vi "RT Main.vi"() -> ()   [LabVIEW 2015]
uses:
  Controls/RT controls.ctl
panel:
  in  "Under":bool
  in  "Break":bool
  in  "Enum":enum16{"3rd", "2nd", "1st", "N", "R"}(ring)=enum."R"
  in  "Right":bool
  in  "Left":bool
  in  "Headlights":bool
  in  "Gas":bool
  in  "Keyin":bool
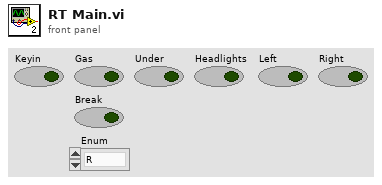
[diagram p1: front panel]
types:
  T1 = typedef "RT controls.ctl" = cluster{"PWM width":dbl, "Headlights":bool, "Red Lights":bool, "Left Turn Lights":bool, "Steer Position":dbl, "Right Turn Lights":bool, "Under Lights":bool}
  T2 = typedef "DIO.lvlib/DIO Reference.ctl" = cluster{"myRIO Reference":T3, "DIO Channels List":T7}
  T3 = typedef "myRIO Generic Hardware Reference.ctl" = cluster{"myRIO Model":T4, "myRIO Hardware Reference":T5}
  T4 = typedef "Hardware Version Enum.ctl" = enum16{"Unknown", "myRIO-1900", "myRIO-1950", "roboRIO"}
  T5 = typedef "myRIO v1.0 Reference.ctl" = cluster{"Generic FPGA Reference":T6, "Allow multiple opens":bool}
  T6 = typedef "Generic FPGA Reference.ctl" = refnum<k20>
  T7 = typedef "DIO Channels List.ctl" = T8[]
  T8 = typedef "DIO Channels Enum.ctl" = enum16{"Not Connected", "C/DIO0", "C/DIO1", "C/DIO2", "C/DIO3", "C/DIO4", "C/DIO5", "C/DIO6", "C/DIO7", "A/DIO0", "A/DIO1", "A/DIO2", "A/DIO3", "A/DIO4", "A/DIO5", "A/DIO6", "A/DIO7", "A/DIO8", "A/DIO9", "A/DIO10", "A/DIO11", "A/DIO12", "A/DIO13", "A/DIO14", "A/DIO15", "B/DIO0", "B/DIO1", "B/DIO2", "B/DIO3", "B/DIO4", "B/DIO5", "B/DIO6", "B/DIO7", "B/DIO8", "B/DIO9", "B/DIO10", "B/DIO11", "B/DIO12", "B/DIO13", "B/DIO14", "B/DIO15", "LED0", "LED1", "LED2", "LED3", "Button0", "DIO/DIO0", "DIO/DIO1", "DIO/DIO2", "DIO/DIO3", "DIO/DIO4", "DIO/DIO5", "DIO/DIO6", "DIO/DIO7", "DIO/DIO8", "DIO/DIO9", "SPI/CS0", "SPI/CS1", "SPI/CS2", "SPI/CS3", "LED RADIO (Green)", "LED RADIO (Red)", "LED COMM (Green)", "LED COMM (Red)", "LED MODE (Green)", "LED MODE (Red)"}
  T9 = typedef "PWM.lvlib/PWM Reference.ctl" = cluster{"myRIO Reference":T3, "PWM Channels Enum":T10, "PWM Configuration":T11}
  T10 = typedef "PWM Channels Enum.ctl" = enum16{"Not Connected", "C/PWM0", "C/PWM1", "A/PWM0", "A/PWM1", "A/PWM2", "B/PWM0", "B/PWM1", "B/PWM2", "PWM/PWM0", "PWM/PWM1", "PWM/PWM2", "PWM/PWM3", "PWM/PWM4", "PWM/PWM5", "PWM/PWM6", "PWM/PWM7", "PWM/PWM8", "PWM/PWM9"}
  T11 = typedef "PWM.lvlib/PWM Configuration.ctl" = cluster{"Frequency":dbl, "Duty Cycle":dbl}
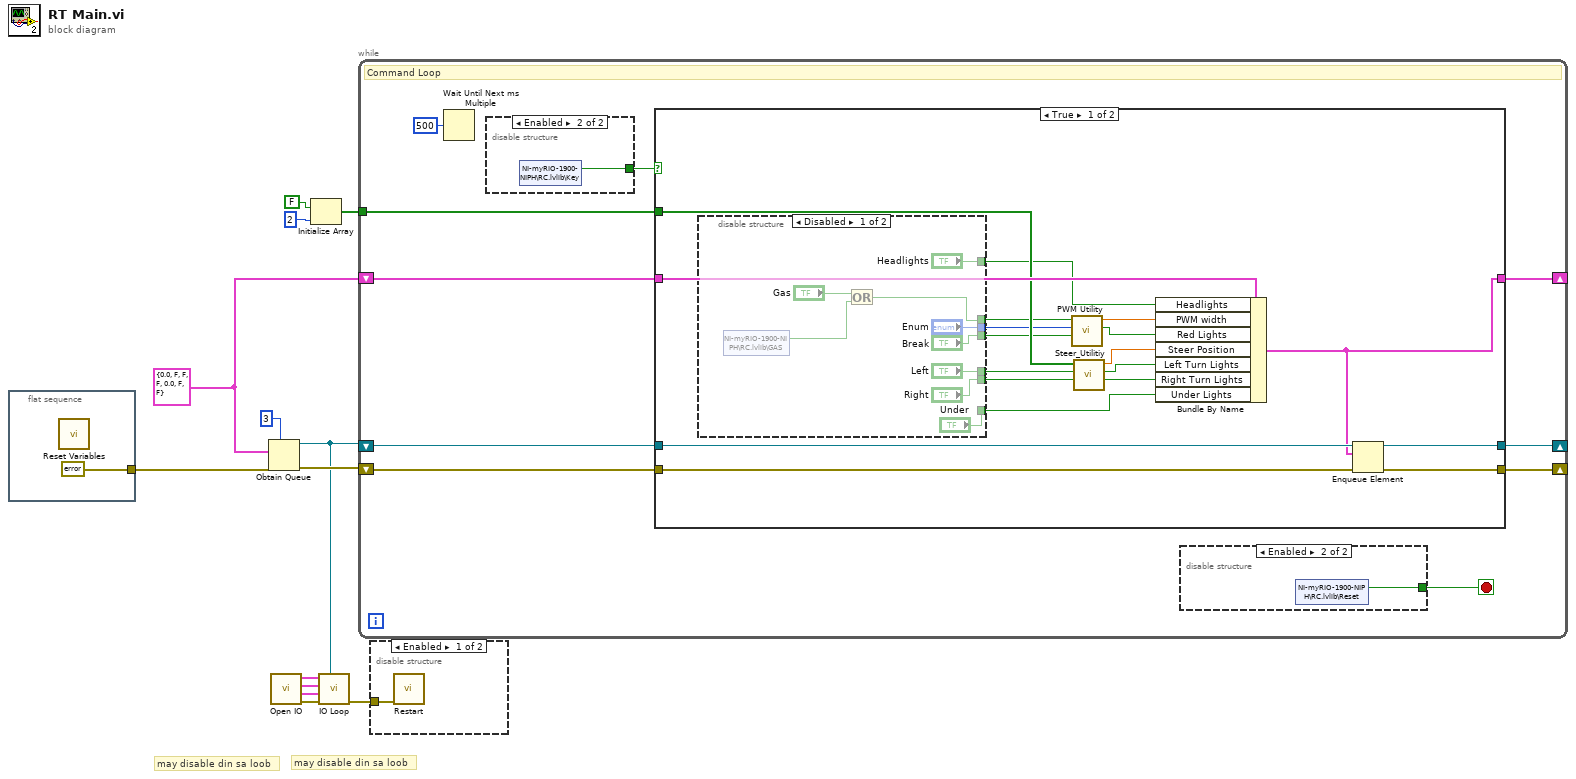
[diagram p0: block diagram]
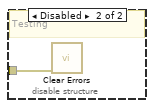
[diagram p2: hidden frame]
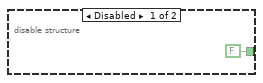
[diagram p3: hidden frame]
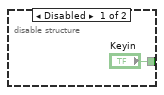
[diagram p4: hidden frame]
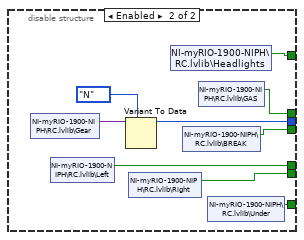
[diagram p5: hidden frame]
diagram:
  w13 = T1 {"PWM width"=0.0, "Headlights"=FALSE, "Red Lights"=FALSE, "Left Turn Lights"=FALSE, "Steer Position"=0.0, "Right Turn Lights"=FALSE, "Under Lights"=FALSE}
  # "may disable din sa loob"
  # "may disable din sa loob"
  n1 = flat-sequence {
    tunnel: [errorcluster {"status"=FALSE, "code"=0, "source"=""} ("error in (no error)")] -> w1
    frame #0 {
      n2 = call "Reset Variables.vi"() -> ()  [unwired: 12 in]
    }
  }
  n3 = Obtain Queue(max queue size (-1, unlimited)=3, element data type=w13, error in (no error)=w1) -> (queue out=w3:refnum<queue>, error out=w8:errorcluster)  [unwired: 2 in, 1 out]
  n4 = call "Open IO.vi"() -> ("error out"=w7:errorcluster, "DIO Ref Out"=w4:T2, "PWM Ref Out"=w5:T9, "PWM Ref Out 2"=w6:T9)  [unwired: 8 in]
  n5 = Initialize Array(FALSE ("Gear UP"), 2 ("dimension size")) -> (w10:bool[])
  n6 = call "IO Loop.vi"("Queue in"=w3, "error in (no error)"=w7, "DIO Ref Out"=w4, "PWM Ref Out"=w5, "PWM Ref Out 2"=w6) -> ("error out"=w2:errorcluster)  [unwired: 6 in]
  n7 = while {
    shift-right: [w21] -> _
    shift-left: w3 -> [w22]
    shift-right: [w19] -> _
    shift-left: w13 -> [w20]
    tunnel: w10 -> [w18]
    shift-right: [w15] -> _
    shift-left: w8 -> [w16]
    stop <- w24 stop-if-true
    # "Command Loop"
    n8 = Wait Until Next ms Multiple(millisecond multiple=u32 500) -> ()  [unwired: 1 out]
    n9 = disable-structure shown="Enabled" {
      disable-tunnel: ["Keyin" w28] -> w23
      frame Disabled {
      }
      frame Enabled {
        n10 = shared-variable "NI-myRIO-1900-NIPH\\RC.lvlib\\Key"() -> (w28:bool)  [unwired: 1 in, 1 out]
      }
    }
    n11 = case shown="True" w23 {
      tunnel: w22 -> [w47 w68]
      tunnel: [w46 w68] -> w21
      tunnel: w20 -> [w45 w67]
      tunnel: [w44 w67] -> w19
      tunnel: w18 -> [w40 _]
      tunnel: w16 -> [w33 w66]
      tunnel: [w32 w66] -> w15
      frame True {
        n12 = disable-structure shown="Disabled" {
          disable-tunnel: ["Right" w65] -> w42
          disable-tunnel: ["Left" w64] -> w41
          disable-tunnel: [w49 w62] -> w38
          disable-tunnel: ["Headlights" w63] -> w34
          disable-tunnel: ["Enum" w58] -> w31
          disable-tunnel: ["Break" w61] -> w30
          disable-tunnel: ["Under" w57] -> w29
          frame Disabled {
            n13 = shared-variable "NI-myRIO-1900-NIPH\\RC.lvlib\\GAS"() -> (w51:bool)  [unwired: 1 in, 1 out]
            n14 = Or(x="Gas", y=w51) -> (x .or. y?=w49:bool)
          }
          frame Enabled {
            n15 = shared-variable "NI-myRIO-1900-NIPH\\RC.lvlib\\Gear"() -> (w60:variant)  [unwired: 1 in, 1 out]
            n16 = shared-variable "NI-myRIO-1900-NIPH\\RC.lvlib\\Left"() -> (w64:bool)  [unwired: 1 in, 1 out]
            n17 = Variant To Data(type=enum16{"3rd", "2nd", "1st", "N", "R"}."N" ("Enum"), Variant=w60) -> (data=w58:enum16{"3rd", "2nd", "1st", "N", "R"})  [unwired: 1 in, 1 out]
            n18 = shared-variable "NI-myRIO-1900-NIPH\\RC.lvlib\\Right"() -> (w65:bool)  [unwired: 1 in, 1 out]
            n19 = shared-variable "NI-myRIO-1900-NIPH\\RC.lvlib\\Headlights"() -> (w63:bool)  [unwired: 1 in, 1 out]
            n20 = shared-variable "NI-myRIO-1900-NIPH\\RC.lvlib\\BREAK"() -> (w61:bool)  [unwired: 1 in, 1 out]
            n21 = shared-variable "NI-myRIO-1900-NIPH\\RC.lvlib\\GAS"() -> (w62:bool)  [unwired: 1 in, 1 out]
            n22 = shared-variable "NI-myRIO-1900-NIPH\\RC.lvlib\\Under"() -> (w57:bool)  [unwired: 1 in, 1 out]
          }
        }
        n23 = call "PWM Utility.vi"("Break"=w30, "Enum"=w31, "GAS"=w38) -> ("Red Lights"=w43:bool, "PWM Width"=w35:dbl)  [unwired: 7 in]
        n24 = call "Steer_Utilitiy.vi"("Right"=w42, "Left"=w41, "array"=w40) -> ("Right"=w39:bool, "Left"=w36:bool, "Steer Position"=w37:dbl)  [unwired: 6 in]
        n25 = Bundle By Name(cluster=w45, "Headlights"=w34, "PWM width"=w35, "Red Lights"=w43, "Steer Position"=w37, "Left Turn Lights"=w36, "Right Turn Lights"=w39, "Under Lights"=w29) -> (w44:T1)
        n26 = Enqueue Element(queue=w47, element=w44, error in (no error)=w33) -> (queue out=w46:refnum<queue>, error out=w32:errorcluster)  [unwired: 1 in, 1 out]
      }
      frame False {
      }
    }
    n27 = disable-structure shown="Enabled" {
      disable-tunnel: [FALSE w26] -> w24
      frame Disabled {
      }
      frame Enabled {
        n28 = shared-variable "NI-myRIO-1900-NIPH\\RC.lvlib\\Reset"() -> (w26:bool)  [unwired: 1 in, 1 out]
      }
    }
  }
  n29 = disable-structure shown="Enabled" {
    disable-tunnel: w2 -> [w69 w70]
    frame Enabled {
      n30 = call "Restart.vi"("error in (no error)"=w69) -> ()  [unwired: 11 in]
    }
    frame Disabled {
      # "Testing"
      n31 = call <vilib>:"Clear Errors.vi"("error in (no error)"=w70) -> ()  [unwired: 5 in, 2 out]
    }
  }
